vi "Read TDMS Comments.vi"(8 "error in (no error)":errorcluster, 10 "path":path, 11 "LVtoITX in":refnum<class "LVtoITX.lvclass">) -> (0 "error out":errorcluster, 2 "Comments":string, 3 "LVtoITX out":refnum<class "LVtoITX.lvclass">)   [LabVIEW 2016, in "LVtoITX.lvclass"]
uses:
  LVtoITX.lvclass
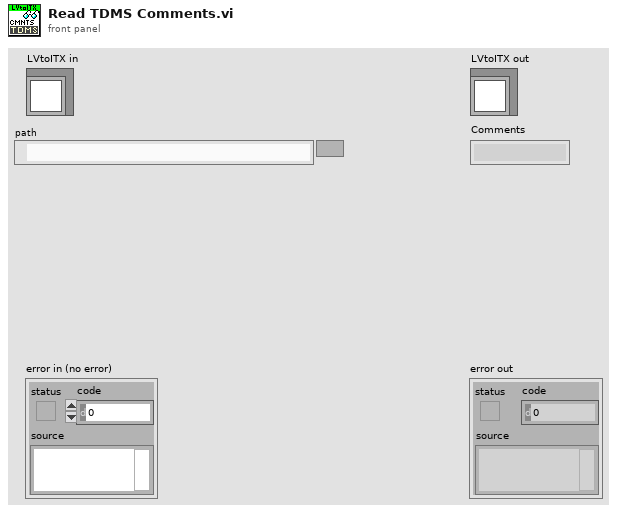
[diagram p1: front panel]
types:
  T1 = enum16{"open", "open or create", "create or replace", "create", "open (read-only)"}
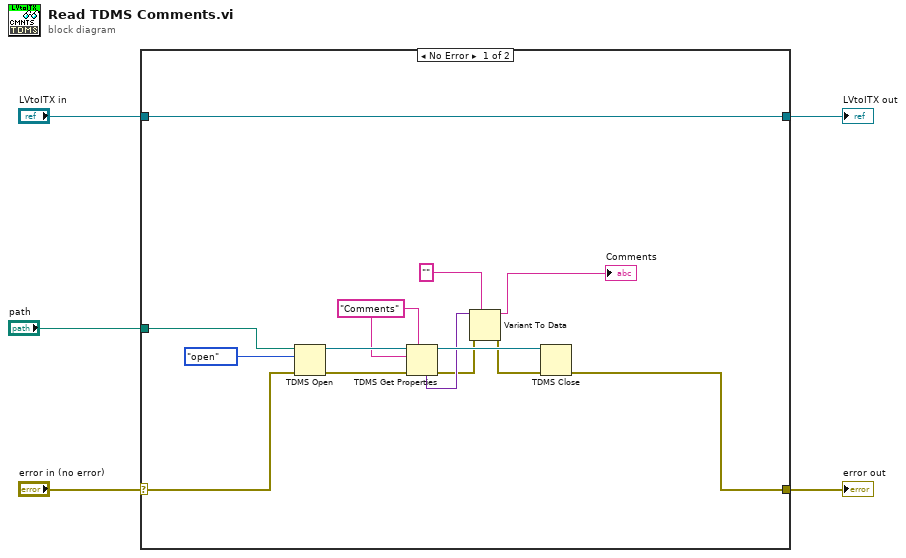
[diagram p0: block diagram]
diagram:
  n1 = case shown="No Error" "error in (no error)" {
    selector: "error in (no error)" -> [w13 w20]
    tunnel: [w16 w20] -> w2
    tunnel: [w12 w21] -> w3
    tunnel: "LVtoITX in" -> [w12 w21]
    tunnel: "path" -> [w15 _]
    frame No Error {
      w11 = "Comments" ("group name")
      n2 = TDMS Open(8:w13, 10:T1."open" ("operation (0:open)"), 11:w15) -> (0:w17:errorcluster, 3:w18:refnum<k34>)  [unwired: 4 in]
      n3 = TDMS Get Properties(7:w11, 8:w17, 10:w11, 11:w18) -> (0:w7:errorcluster, 3:w14:refnum<k34>, 4:w10:variant)  [unwired: 2 in, 3 out]
      n4 = Variant To Data(error in=w7, type="" ("group name"), Variant=w10) -> (data=→"Comments":string, error out=w6:errorcluster)
      n5 = TDMS Close(8:w6, 11:w14) -> (0:w16:errorcluster)  [unwired: 1 out]
    }
    frame Error {
    }
  }
  "error out" <- w2
  "LVtoITX out" <- w3
